vi "Events.vi"(11 "Control in":refnum<class "Control.lvclass">) -> (2 "Events":T1[](array[typedef]))   [LabVIEW 2020, in "VolatusGUI.lvlib" / "Control.lvclass"]
uses:
  Control.lvclass
  Control.lvclass/Control.ctl
  Control Event Registrations/Control Event Registrations.lvclass
  Control Event.ctl
  VolatusGUI.lvlib
  Event Registration.ctl
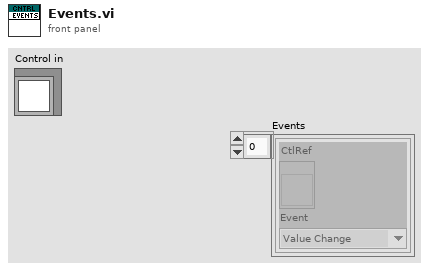
[diagram p1: front panel]
types:
  T1 = typedef "VolatusGUI.lvlib/Event Registration.ctl" = cluster{"CtlRef":refnum<vi>, "Event":T2}
  T2 = typedef "VolatusGUI.lvlib/Control Event.ctl" = enum16{"Value Change", "Shortcut Menu"}
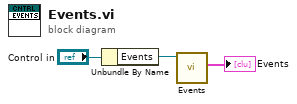
[diagram p0: block diagram]
diagram:
  n1 = Unbundle By Name("Control in") -> ("Events"=w2:refnum<class "Control Event Registrations.lvclass">)
  n2 = call "Events.vi"("Control Event Registrations in"=w2) -> ("Events"=→"Events":T1[])  [unwired: 10 in]
